vi "sub vi - calibration v2.vi"(6 "Samples":dbl, 8 "Task2":dbl, 9 "Task1":dbl, 10 "Task0":dbl, 11 "Temp Test Cal":dbl) -> ()   [LabVIEW 2017]
uses:
  <vilib>/Platform/TimedLoop/XDataNode/timing_clust.ctl
  <vilib>/Platform/TimedLoop/XDataNode/nitl_modes.ctl
  <vilib>/Platform/TimedLoop/XDataNode/wakeup.ctl
  <vilib>/platform/TimedLoop/XDataNode/XDataNode.xnode
  <vilib>/Platform/TimedLoop/XDataNode/XDNodeRunTimeDep.lvlib
panel:
  out "UPDATE":bool
  in  "stop":bool
  in  "Tab Control":T1(tab)
  out "1-2(TN) Run":dbl
  out "1-2(TL) Run":dbl
  out "1-1(TN) Run":dbl
  out "1-1(TL) Run":dbl
  out "LAB01-1 (GRAPH)":dynamicdata(graph)
  out "LAB01-2 (GRAPH)":dynamicdata(graph)
  in  "LAB01 (CAL)":T2 {"2 (TN) cal" min=0.0 step=0.01 format="%.2f"; "2 (TL) cal" min=0.0 step=0.01 format="%.2f"; "2 (PF) cal" min=0.0 step=0.01 format="%.2f"; "2 (V) cal" min=0.0 step=0.01 format="%.2f"; "2 (A) cal" min=0.0 step=0.01 format="%.2f"; "1 (TN) cal" min=0.0 step=0.01 format="%.2f"; "1 (TL) cal" min=0.0 step=0.01 format="%.2f"; "1 (PF) cal" min=0.0 step=0.01 format="%.2f"; "1 (V) cal" min=0.0 step=0.01 format="%.2f"; "1  (A) cal" min=0.0 step=0.01 format="%.2f"}
  out "LAB01 (SIGNALS)":T3 {"2 (PF)" format="%.2f"; "2 (A)" format="%.1f"; "1 (PF)" format="%.2f"; "1 (A)" format="%.1f"}
  out "2-2(TN) Run":dbl
  out "2-2(TL) Run":dbl
  out "2-1(TN) Run":dbl
  out "2-1(TL) Run":dbl
  out "LAB02 (SIGNALS)":T3 {"2 (PF)" format="%.2f"; "2 (A)" format="%.1f"; "1 (PF)" format="%.2f"; "1 (A)" format="%.1f"}
  in  "LAB02 (CAL)":T4 {"2 (TN) cal" min=0.0 step=0.01 format="%.2f"; "2 (TL) cal" min=0.0 step=0.01 format="%.2f"; "2 (PF) cal" min=0.0 step=0.01 format="%.2f"; "2 (V) cal" min=0.0 step=0.01 format="%.2f"; "2 (A) cal" min=0.0 step=0.01 format="%.2f"; "1 (TN) cal" min=0.0 step=0.01 format="%.2f"; "1 (TL) cal" min=0.0 step=0.01 format="%.2f"; "1 (PF) cal" min=0.0 step=0.01 format="%.2f"; "1 (V) cal" min=0.0 step=0.01 format="%.2f"; "1 (A) cal" min=0.0 step=0.01 format="%.2f"}
  out "LAB02-2 (GRAPH)":dynamicdata(graph)
  out "LAB02-1 (GRAPH)":dynamicdata(graph)
  out "3-2(TN) Run":dbl
  out "3-2(TL) Run":dbl
  out "3-1(TN) Run":dbl
  out "3-1(TL) Run":dbl
  out "LAB03 (SIGNALS)":T3 {"2 (PF)" format="%.2f"; "2 (A)" format="%.1f"; "1 (PF)" format="%.2f"; "1 (A)" format="%.1f"}
  in  "LAB03 (CAL)":T2 {"2 (TN) cal" min=0.0 step=0.01 format="%.2f"; "2 (TL) cal" min=0.0 step=0.01 format="%.2f"; "2 (PF) cal" min=0.0 step=0.01 format="%.2f"; "2 (V) cal" min=0.0 step=0.01 format="%.2f"; "2 (A) cal" min=0.0 step=0.01 format="%.2f"; "1 (TN) cal" min=0.0 step=0.01 format="%.2f"; "1 (TL) cal" min=0.0 step=0.01 format="%.2f"; "1 (PF) cal" min=0.0 step=0.01 format="%.2f"; "1 (V) cal" min=0.0 step=0.01 format="%.2f"; "1  (A) cal" min=0.0 step=0.01 format="%.2f"}
  out "LAB03-2 (GRAPH)":dynamicdata(graph)
  out "LAB03-1 (GRAPH)":dynamicdata(graph)
  out "4-2(TN) Run":dbl
  out "4-2(TL) Run":dbl
  out "4-1(TN) Run":dbl
  out "4-1(TL) Run":dbl
  out "LAB04 (SIGNALS)":T3 {"2 (PF)" format="%.2f"; "2 (A)" format="%.1f"; "1 (PF)" format="%.2f"; "1 (A)" format="%.1f"}
  in  "LAB04 (CAL)":T2 {"2 (TN) cal" min=0.0 step=0.01 format="%.2f"; "2 (TL) cal" min=0.0 step=0.01 format="%.2f"; "2 (PF) cal" min=0.0 step=0.01 format="%.2f"; "2 (V) cal" min=0.0 step=0.01 format="%.2f"; "2 (A) cal" min=0.0 step=0.01 format="%.2f"; "1 (TN) cal" min=0.0 step=0.01 format="%.2f"; "1 (TL) cal" min=0.0 step=0.01 format="%.2f"; "1 (PF) cal" min=0.0 step=0.01 format="%.2f"; "1 (V) cal" min=0.0 step=0.01 format="%.2f"; "1  (A) cal" min=0.0 step=0.01 format="%.2f"}
  out "LAB04-2 (GRAPH)":dynamicdata(graph)
  out "LAB04-1 (GRAPH)":dynamicdata(graph)
  out "5-2(TN) Run":dbl
  out "5-2(TL) Run":dbl
  out "5-1(TN) Run":dbl
  out "5-1(TL) Run":dbl
  out "LAB05 (SIGNALS)":T3 {"2 (PF)" format="%.2f"; "2 (A)" format="%.1f"; "1 (PF)" format="%.2f"; "1 (A)" format="%.1f"}
  in  "LAB05 (CAL)":T2 {"2 (TN) cal" min=0.0 step=0.01 format="%.2f"; "2 (TL) cal" min=0.0 step=0.01 format="%.2f"; "2 (PF) cal" min=0.0 step=0.01 format="%.2f"; "2 (V) cal" min=0.0 step=0.01 format="%.2f"; "2 (A) cal" min=0.0 step=0.01 format="%.2f"; "1 (TN) cal" min=0.0 step=0.01 format="%.2f"; "1 (TL) cal" min=0.0 step=0.01 format="%.2f"; "1 (PF) cal" min=0.0 step=0.01 format="%.2f"; "1 (V) cal" min=0.0 step=0.01 format="%.2f"; "1  (A) cal" min=0.0 step=0.01 format="%.2f"}
  out "LAB05-2 (GRAPH)":dynamicdata(graph)
  out "LAB05-1 (GRAPH)":dynamicdata(graph)
  in  "TEMP REF cal":dbl
  out "AMBIENT TEMP REF":dbl format="%.1f"
  out "Data2":waveform(dbl)[](graph)
  out "Data1":waveform(dbl)[](graph)
  out "Data0":waveform(dbl)[](graph)
  out "Analog Loop Time":dbl
  out "Temperature data error":bool
  out "file error out":errorcluster
  out "AI Error":errorcluster[](array[cluster])
  out "data 0":waveform(dbl)[](array[waveform])
  out "data 1":waveform(dbl)[](array[waveform])
  out "data 2":waveform(dbl)[](array[waveform])
  # "This value is only applied during\ntesting to adjust for insulatred probe\nprofile during current flow temp rise.\nIf any change is made here, make sure\nvalue is changed to same value on\nADM tab."
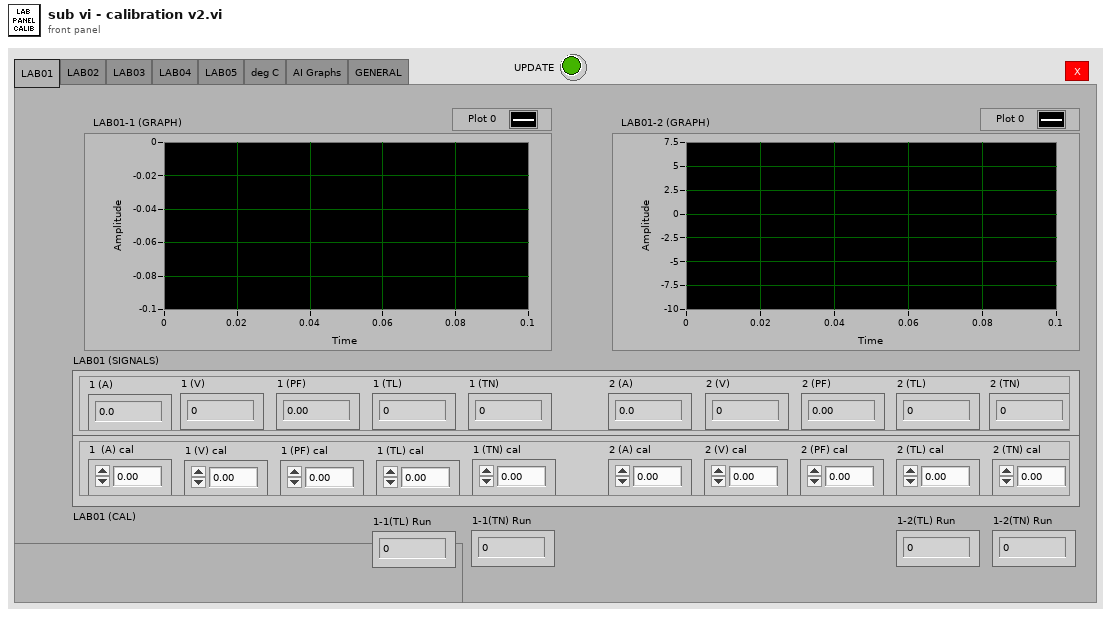
[diagram p1: front panel]
types:
  T1 = enum32{"LAB01", "LAB02", "LAB03", "LAB04", "LAB05", "deg C", "AI Graphs", "GENERAL"}
  T2 = cluster{"1  (A) cal":dbl, "1 (V) cal":dbl, "1 (PF) cal":dbl, "1 (TL) cal":dbl, "1 (TN) cal":dbl, "2 (A) cal":dbl, "2 (V) cal":dbl, "2 (PF) cal":dbl, "2 (TL) cal":dbl, "2 (TN) cal":dbl}
  T3 = cluster{"1 (TL)":dbl, "1 (TN)":dbl, "2 (TL)":dbl, "2 (TN)":dbl, "1 (A)":dbl, "1 (V)":dbl, "1 (PF)":dbl, "2 (A)":dbl, "2 (V)":dbl, "2 (PF)":dbl}
  T4 = cluster{"1 (A) cal":dbl, "1 (V) cal":dbl, "1 (PF) cal":dbl, "1 (TL) cal":dbl, "1 (TN) cal":dbl, "2 (A) cal":dbl, "2 (V) cal":dbl, "2 (PF) cal":dbl, "2 (TL) cal":dbl, "2 (TN) cal":dbl}
  T5 = enum16{"open", "replace", "create", "open or create", "replace or create", "replace or create with confirmation"}
  T6 = typedef "XDNodeRunTimeDep.lvlib/timing_clust.ctl" = cluster{"Expected End [f-1]":u64, "Actual End [f-1]":u64, "Finished Late? [f-1]":bool, "Expected End [i-1]":u64, "Actual End [i-1]":u64, "Finished Late? [i-1]":bool, "Expected Start [i]":u64, "Actual Start [i]":u64, "Expected Start [f]":u64, "Actual Start [f]":u64, "Source Name":string, "Structure Name":string, "Period":i64, "Deadline":i64, "Offset":i64, "Start":i64, "Priority":i32, "Timeout":i32, "Mode":T7, "Wakeup Reason":T8, "Error":errorcluster, "Source Type":string, "Secondary Source Type":string, "Global End Time":u64, "Global Start Time":u64, "Frame Duration":u64, "Iteration Duration":u64, "Assigned CPU":i32, "I/O Scan Engine Mode":u32}
  T7 = typedef "XDNodeRunTimeDep.lvlib/nitl_modes.ctl" = enum32{"No Change", "Process missed periods, maintain original phase", "Discard missed periods, maintain original phase", "Process missed periods, ignore original phase", "Discard missed periods, ignore original phase"}
  T8 = typedef "XDNodeRunTimeDep.lvlib/wakeup.ctl" = enum32{"Normal", "Aborted", "Asynchronous wakeup", "Timing source error", "Timed loop error", "Timeout"}
  T9 = cluster{"LAB01-1 (A)":dbl, "LAB01-1 (V)":dbl, "LAB01-1 (PF)":dbl, "LAB01-2 (A)":dbl, "LAB01-2 (V)":dbl, "LAB01-2 (PF)":dbl}
  T10 = cluster{"LAB02-1 (A)":dbl, "LAB02-1 (V)":dbl, "LAB02-1 (PF)":dbl, "LAB02-2 (A)":dbl, "LAB02-2 (V)":dbl, "LAB02-2 (PF)":dbl}
  T11 = cluster{"LAB03-1 (A)":dbl, "LAB03-1 (V)":dbl, "LAB03-1 (PF)":dbl, "LAB03-2 (A)":dbl, "LAB03-2 (V)":dbl, "LAB03-2 (PF)":dbl}
  T12 = cluster{"LAB04-1 (A)":dbl, "LAB04-1 (V)":dbl, "LAB04-1 (PF)":dbl, "LAB04-2 (A)":dbl, "LAB04-2 (V)":dbl, "LAB04-2 (PF)":dbl}
  T13 = cluster{"LAB05-1 (A)":dbl, "LAB05-1 (V)":dbl, "LAB05-1 (PF)":dbl, "LAB05-2 (A)":dbl, "LAB05-2 (V)":dbl, "LAB05-2 (PF)":dbl}
  T14 = cluster{"T1":dbl, "T2":dbl, "T3":dbl, "T4":dbl, "ID":dbl, "ER":dbl}
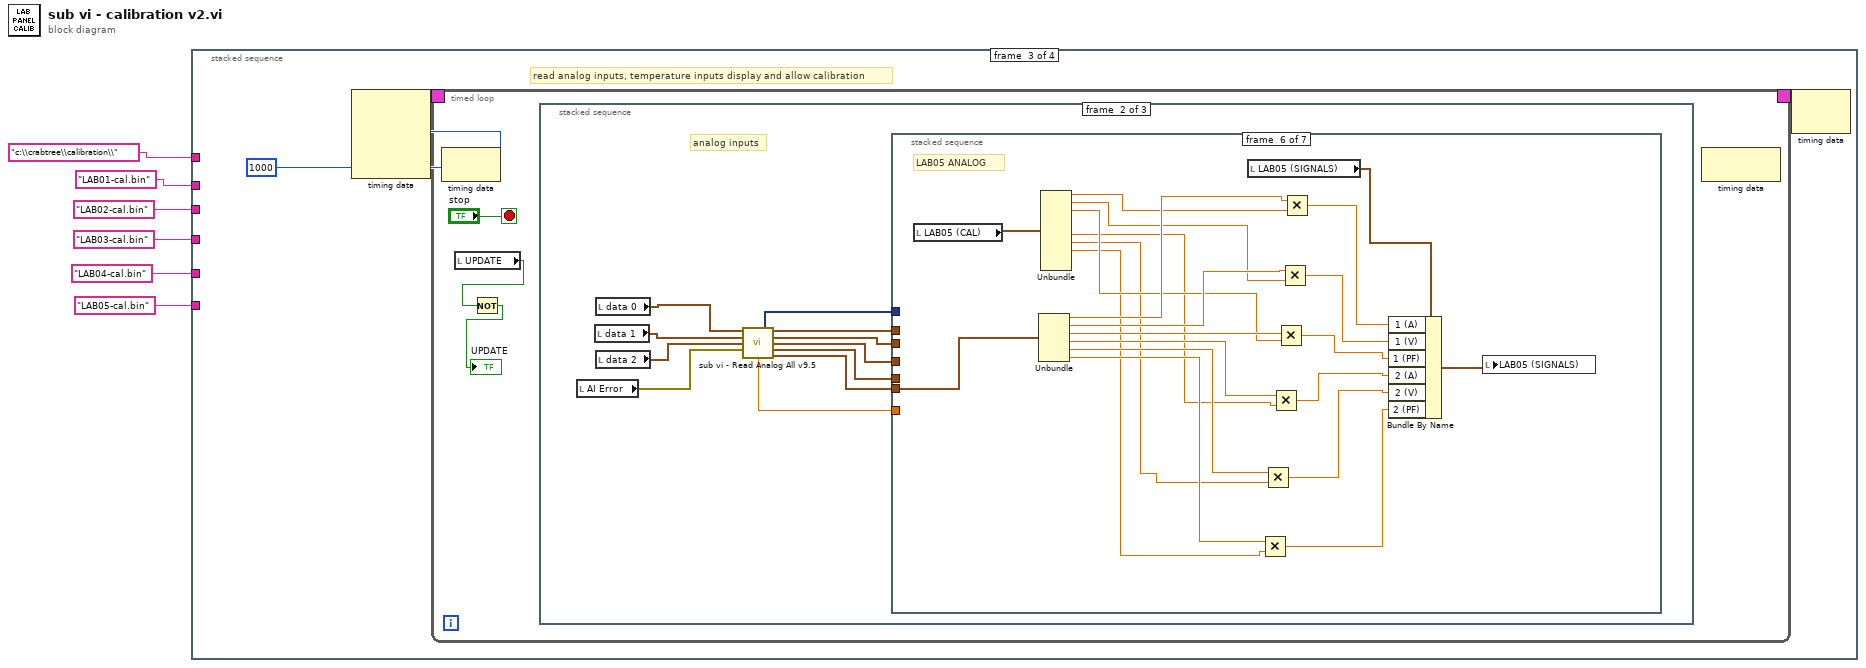
[diagram p0: block diagram]
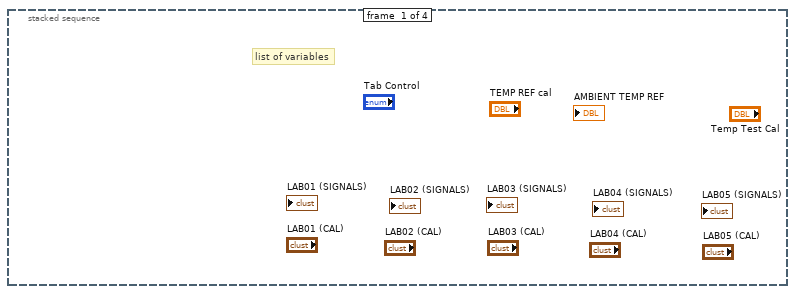
[diagram p2: hidden frame]
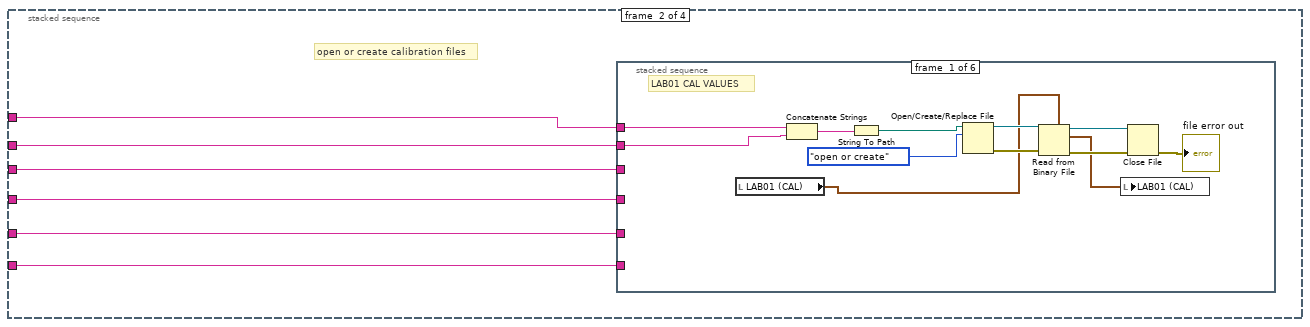
[diagram p3: hidden frame]
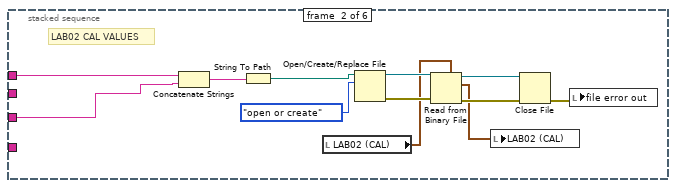
[diagram p4: hidden frame]
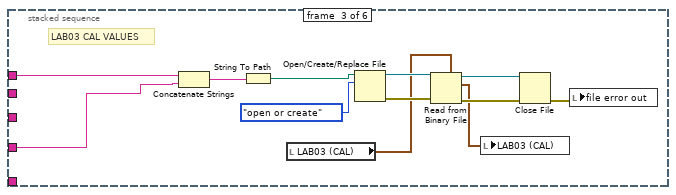
[diagram p5: hidden frame]
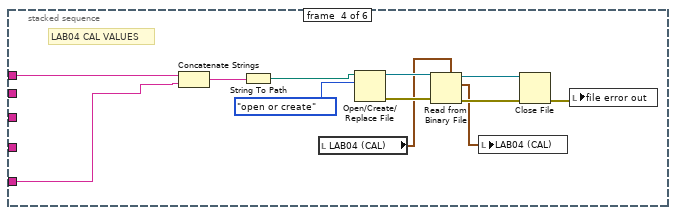
[diagram p6: hidden frame]
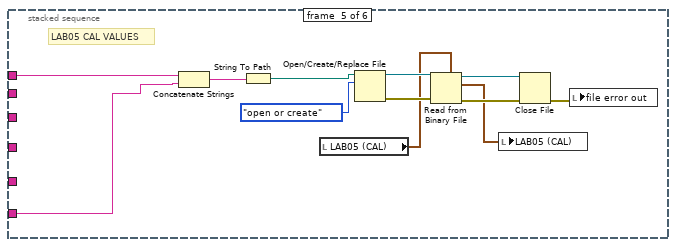
[diagram p7: hidden frame]
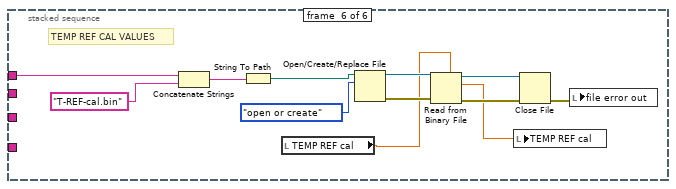
[diagram p8: hidden frame]
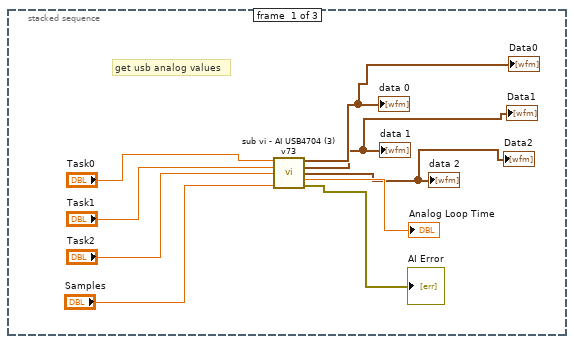
[diagram p9: hidden frame]
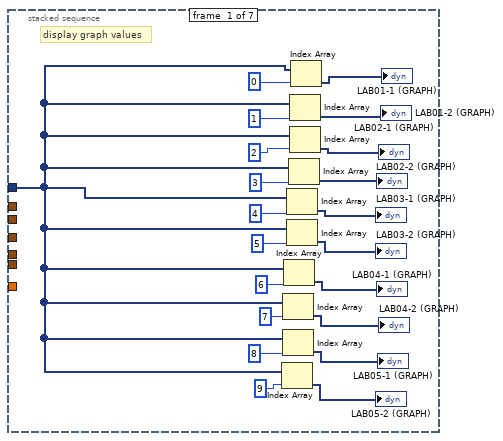
[diagram p10: hidden frame]
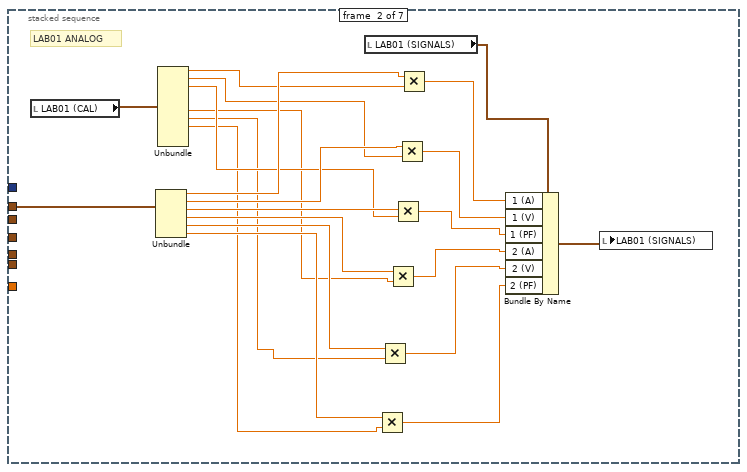
[diagram p11: hidden frame]
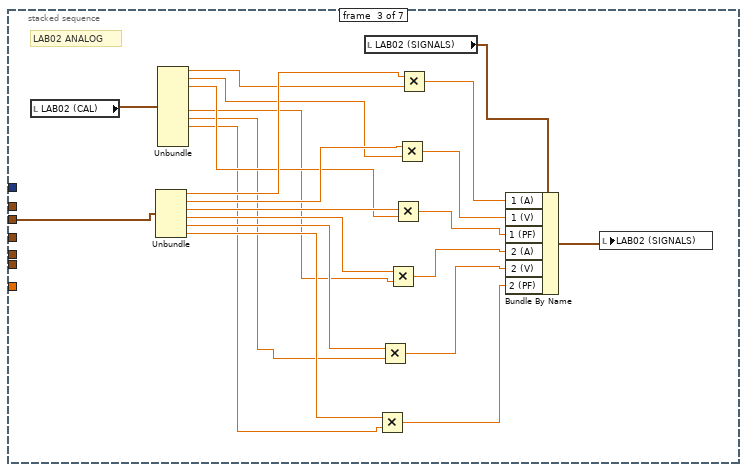
[diagram p12: hidden frame]
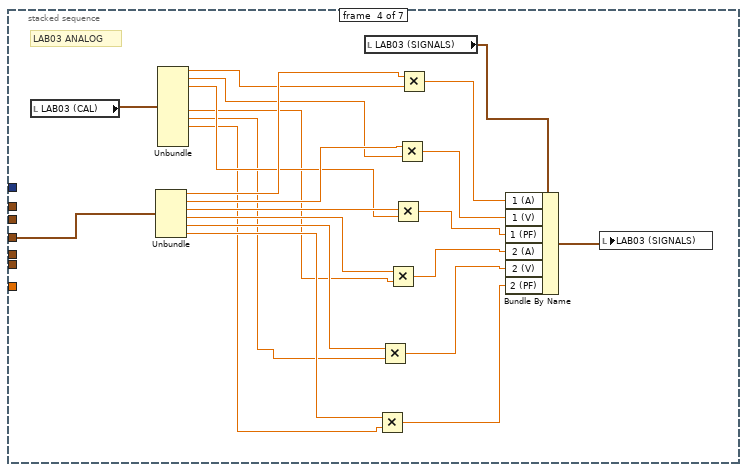
[diagram p13: hidden frame]
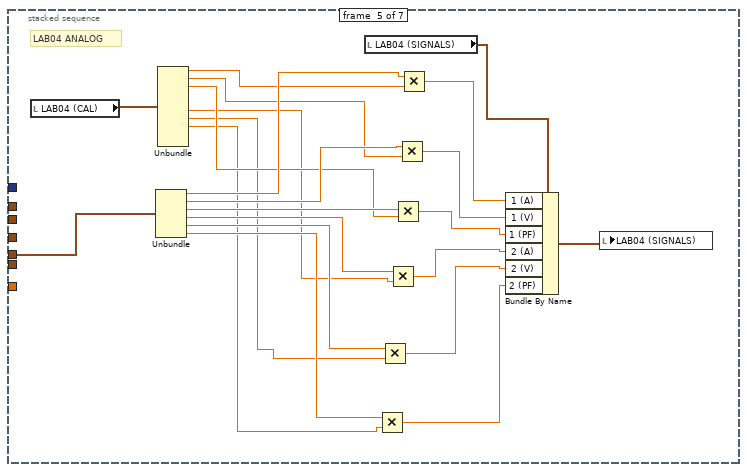
[diagram p14: hidden frame]
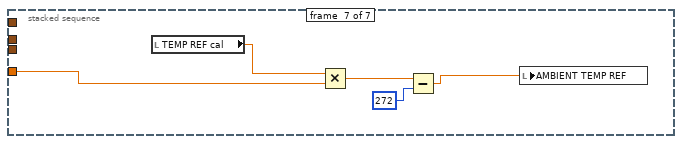
[diagram p15: hidden frame]
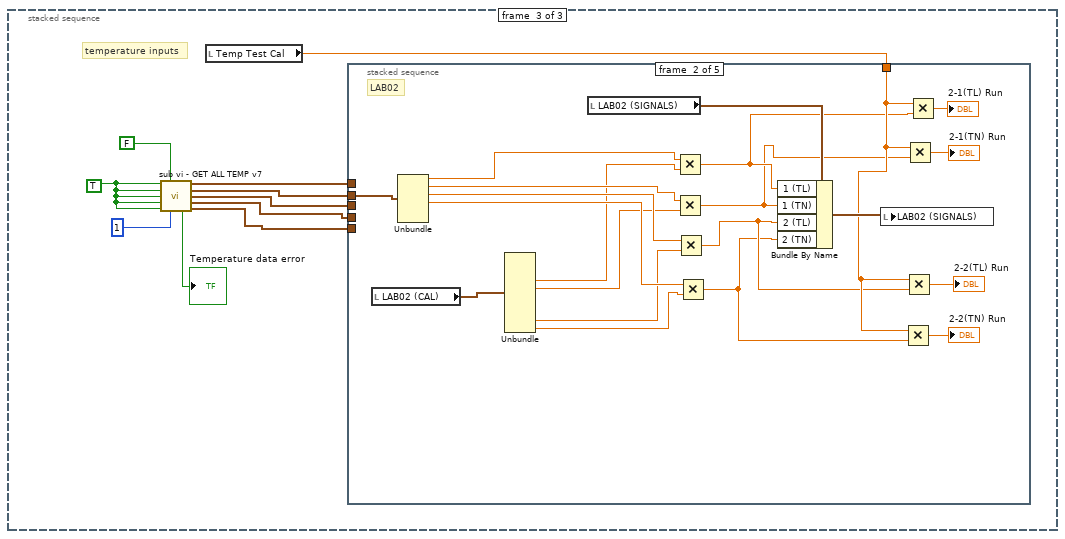
[diagram p16: hidden frame]
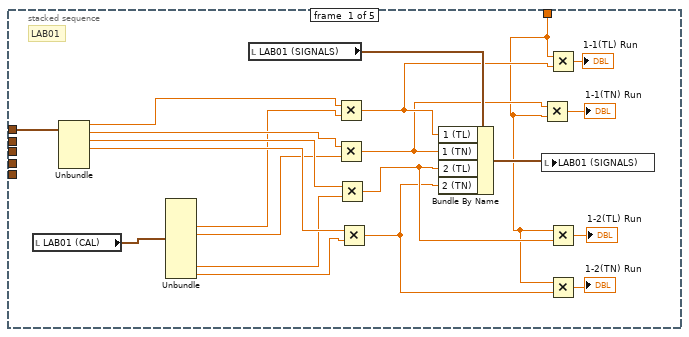
[diagram p17: hidden frame]
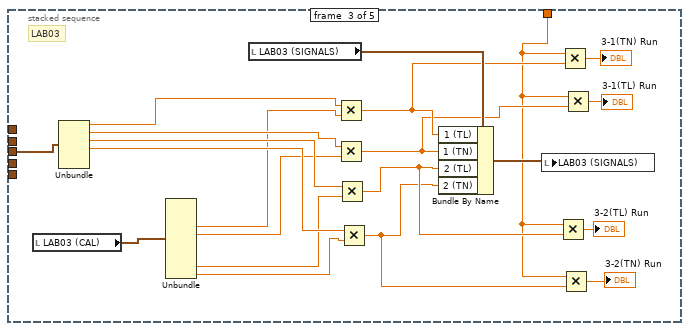
[diagram p18: hidden frame]
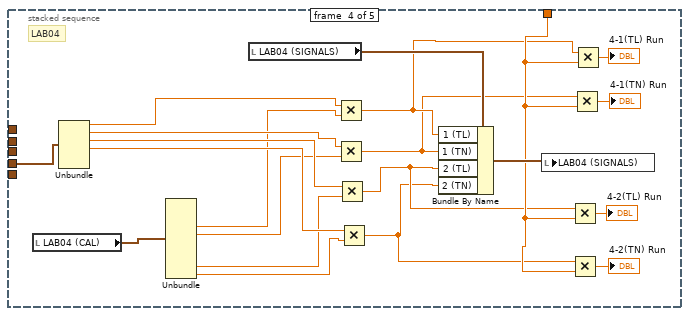
[diagram p19: hidden frame]
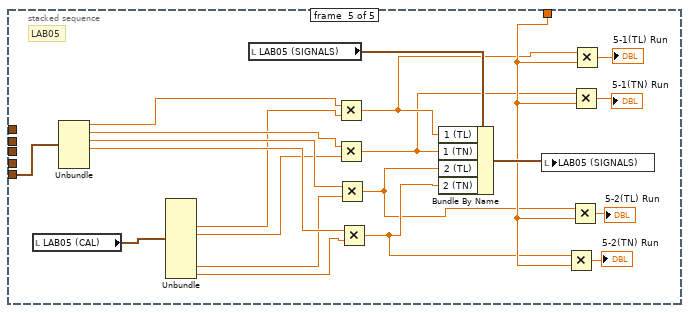
[diagram p20: hidden frame]
diagram:
  n1 = stacked-sequence {
    tunnel: "c:\\crabtree\\calibration\\" -> [_ w12 _ w373]
    tunnel: "LAB01-cal.bin" -> [_ w11 _ w372]
    tunnel: "LAB02-cal.bin" -> [_ w10 _ w371]
    tunnel: "LAB03-cal.bin" -> [_ w9 _ w370]
    tunnel: "LAB04-cal.bin" -> [_ w8 _ w369]
    tunnel: "LAB05-cal.bin" -> [_ w7 _ w368]
    frame #0 {
      # "list of variables"
    }
    frame #1 {
      # "open or create calibration files"
      n2 = stacked-sequence {
        tunnel: w12 -> [w24 w36 w48 w60 w72 w84]
        tunnel: w11 -> [w15 _ _ _ _ _]
        tunnel: w10 -> [_ w27 _ _ _ _]
        tunnel: w9 -> [_ _ w39 _ _ _]
        tunnel: w8 -> [_ _ _ w52 _ _]
        tunnel: w7 -> [_ _ _ _ w63 _]
        frame #0 {
          # "LAB01 CAL VALUES"
          n3 = local read "LAB01 (CAL)"() -> (w14:T2)
          n4 = Concatenate Strings(w24, w15) -> (w23:string)
          n5 = String To Path(string=w23) -> (path=w22:path)
          n6 = Open/Create/Replace File(file path (use dialog)=w22, operation (0:open)=T5."open or create") -> (refnum out=w21:refnum<file>, error out=w20:errorcluster)  [unwired: 4 in, 1 out]
          n7 = Read from Binary File(5:w14, 8:w20, 11:w21) -> (0:w18:errorcluster, 2:w13:T2, 3:w19:refnum<file>)  [unwired: 3 in, 1 out]
          n8 = local write "LAB01 (CAL)"(w13) -> ()
          n9 = Close File(refnum=w19, error in=w18) -> (error out=→"file error out":errorcluster)  [unwired: 1 out]
        }
        frame #1 {
          # "LAB02 CAL VALUES"
          n10 = Concatenate Strings(w36, w27) -> (w35:string)
          n11 = String To Path(string=w35) -> (path=w34:path)
          n12 = local read "LAB02 (CAL)"() -> (w26:T4)
          n13 = Open/Create/Replace File(file path (use dialog)=w34, operation (0:open)=T5."open or create") -> (refnum out=w33:refnum<file>, error out=w32:errorcluster)  [unwired: 4 in, 1 out]
          n14 = Read from Binary File(5:w26, 8:w32, 11:w33) -> (0:w30:errorcluster, 2:w25:T4, 3:w31:refnum<file>)  [unwired: 3 in, 1 out]
          n15 = local write "LAB02 (CAL)"(w25) -> ()
          n16 = Close File(refnum=w31, error in=w30) -> (error out=w28:errorcluster)  [unwired: 1 out]
          n17 = local write "file error out"(w28) -> ()
        }
        frame #2 {
          # "LAB03 CAL VALUES"
          n18 = Concatenate Strings(w48, w39) -> (w47:string)
          n19 = String To Path(string=w47) -> (path=w46:path)
          n20 = local read "LAB03 (CAL)"() -> (w38:T2)
          n21 = Open/Create/Replace File(file path (use dialog)=w46, operation (0:open)=T5."open or create") -> (refnum out=w45:refnum<file>, error out=w44:errorcluster)  [unwired: 4 in, 1 out]
          n22 = Read from Binary File(5:w38, 8:w44, 11:w45) -> (0:w42:errorcluster, 2:w37:T2, 3:w43:refnum<file>)  [unwired: 3 in, 1 out]
          n23 = local write "LAB03 (CAL)"(w37) -> ()
          n24 = Close File(refnum=w43, error in=w42) -> (error out=w40:errorcluster)  [unwired: 1 out]
          n25 = local write "file error out"(w40) -> ()
        }
        frame #3 {
          # "LAB04 CAL VALUES"
          n26 = Concatenate Strings(w60, w52) -> (w59:string)
          n27 = String To Path(string=w59) -> (path=w58:path)
          n28 = local read "LAB04 (CAL)"() -> (w50:T2)
          n29 = Open/Create/Replace File(file path (use dialog)=w58, operation (0:open)=T5."open or create") -> (refnum out=w57:refnum<file>, error out=w56:errorcluster)  [unwired: 4 in, 1 out]
          n30 = Read from Binary File(5:w50, 8:w56, 11:w57) -> (0:w54:errorcluster, 2:w49:T2, 3:w55:refnum<file>)  [unwired: 3 in, 1 out]
          n31 = local write "LAB04 (CAL)"(w49) -> ()
          n32 = Close File(refnum=w55, error in=w54) -> (error out=w53:errorcluster)  [unwired: 1 out]
          n33 = local write "file error out"(w53) -> ()
        }
        frame #4 {
          # "LAB05 CAL VALUES"
          n34 = Concatenate Strings(w72, w63) -> (w71:string)
          n35 = String To Path(string=w71) -> (path=w70:path)
          n36 = local read "LAB05 (CAL)"() -> (w62:T2)
          n37 = Open/Create/Replace File(file path (use dialog)=w70, operation (0:open)=T5."open or create") -> (refnum out=w69:refnum<file>, error out=w68:errorcluster)  [unwired: 4 in, 1 out]
          n38 = Read from Binary File(5:w62, 8:w68, 11:w69) -> (0:w66:errorcluster, 2:w61:T2, 3:w67:refnum<file>)  [unwired: 3 in, 1 out]
          n39 = local write "LAB05 (CAL)"(w61) -> ()
          n40 = Close File(refnum=w67, error in=w66) -> (error out=w64:errorcluster)  [unwired: 1 out]
          n41 = local write "file error out"(w64) -> ()
        }
        frame #5 {
          # "TEMP REF CAL VALUES"
          n42 = Concatenate Strings(w84, "T-REF-cal.bin") -> (w83:string)
          n43 = String To Path(string=w83) -> (path=w82:path)
          n44 = local read "TEMP REF cal"() -> (w74:dbl)
          n45 = Open/Create/Replace File(file path (use dialog)=w82, operation (0:open)=T5."open or create") -> (refnum out=w81:refnum<file>, error out=w80:errorcluster)  [unwired: 4 in, 1 out]
          n46 = Read from Binary File(5:w74, 8:w80, 11:w81) -> (0:w78:errorcluster, 2:w73:dbl, 3:w79:refnum<file>)  [unwired: 3 in, 1 out]
          n47 = local write "TEMP REF cal"(w73) -> ()
          n48 = Close File(refnum=w79, error in=w78) -> (error out=w76:errorcluster)  [unwired: 1 out]
          n49 = local write "file error out"(w76) -> ()
        }
      }
    }
    frame #2 {
      # "read analog inputs, temperature inputs display and allow calibration"
      n50 = node-c288(1000) -> (w87:T6)  [unwired: 3 in]
      n51 = timed-loop {
        timing: w87 -> [_]
        timing-out: [_] -> w86
        stop <- "stop" stop-if-true
        n52 = node-c288() -> ()  [unwired: 1 in, 1 out]
        n53 = local read "UPDATE"() -> (w88:bool)
        n54 = Not(x=w88) -> (.not. x?=→"UPDATE":bool)
        n55 = stacked-sequence {
          frame #0 {
            # "get usb analog values"
            n56 = call "sub vi - AI USB4704 (3) v73.vi"("Task0"="Task0", "Task1"="Task1", "Task2"="Task2", "SAMPLES"="Samples") -> ("data 0"=→"data 0" →"Data0":waveform(dbl)[], "data 1"=→"data 1" →"Data1":waveform(dbl)[], "data 2"=→"data 2" →"Data2":waveform(dbl)[], "loop time"=→"Analog Loop Time":dbl, "error array"=→"AI Error":errorcluster[])  [unwired: 7 in]
          }
          frame #1 {
            # "analog inputs"
            n57 = local read "AI Error"() -> (w100:errorcluster[])
            n58 = local read "data 1"() -> (w102:waveform(dbl)[])
            n59 = local read "data 0"() -> (w103:waveform(dbl)[])
            n60 = local read "data 2"() -> (w101:waveform(dbl)[])
            n61 = call "sub vi - Read Analog All v9.5.vi"("data 0"=w103, "data 1"=w102, "data 2"=w101, "AI Error"=w100) -> ("array GRAPH"=w110:dynamicdata[], "LAB01"=w109:T9, "LAB02"=w108:T10, "LAB03"=w107:T11, "LAB04"=w106:T12, "deg C"=w104:dbl, "LAB05"=w105:T13)  [unwired: 4 in, 1 out]
            n62 = stacked-sequence {
              tunnel: w110 -> [w130 _ _ _ _ _ _]
              tunnel: w109 -> [_ w152 _ _ _ _ _]
              tunnel: w107 -> [_ _ _ w176 _ _ _]
              tunnel: w108 -> [_ _ w154 _ _ _ _]
              tunnel: w106 -> [_ _ _ _ w198 _ _]
              tunnel: w105 -> [_ _ _ _ _ w220 _]
              tunnel: w104 -> [_ _ _ _ _ _ w245]
              frame #0 {
                # "display graph values"
                n63 = Index Array(array=w130, index=9) -> (element=→"LAB05-2 (GRAPH)":dynamicdata)
                n64 = Index Array(array=w130, index=7) -> (element=→"LAB04-2 (GRAPH)":dynamicdata)
                n65 = Index Array(array=w130, index=8) -> (element=→"LAB05-1 (GRAPH)":dynamicdata)
                n66 = Index Array(array=w130, index=6) -> (element=→"LAB04-1 (GRAPH)":dynamicdata)
                n67 = Index Array(array=w130, index=4) -> (element=→"LAB03-1 (GRAPH)":dynamicdata)
                n68 = Index Array(array=w130, index=5) -> (element=→"LAB03-2 (GRAPH)":dynamicdata)
                n69 = Index Array(array=w130, index=3) -> (element=→"LAB02-2 (GRAPH)":dynamicdata)
                n70 = Index Array(array=w130, index=1) -> (element=→"LAB01-2 (GRAPH)":dynamicdata)
                n71 = Index Array(array=w130, index=2) -> (element=→"LAB02-1 (GRAPH)":dynamicdata)
                n72 = Index Array(array=w130, index=0) -> (element=→"LAB01-1 (GRAPH)":dynamicdata)
              }
              frame #1 {
                # "LAB01 ANALOG"
                n73 = local read "LAB01 (CAL)"() -> (w153:T2)
                n74 = Unbundle(w152) -> ("LAB01-1 (A)"=w151:dbl, "LAB01-1 (V)"=w150:dbl, "LAB01-1 (PF)"=w149:dbl, "LAB01-2 (A)"=w148:dbl, "LAB01-2 (V)"=w147:dbl, "LAB01-2 (PF)"=w146:dbl)
                n75 = Unbundle(w153) -> ("1  (A) cal"=w145:dbl, "1 (V) cal"=w144:dbl, "1 (PF) cal"=w143:dbl, "2 (A) cal"=w142:dbl, "2 (V) cal"=w141:dbl, "2 (PF) cal"=w140:dbl)  [unwired: 4 out]
                n76 = local read "LAB01 (SIGNALS)"() -> (w139:T3)
                n77 = Multiply(x=w146, y=w140) -> (x*y=w133:dbl)
                n78 = Multiply(x=w147, y=w141) -> (x*y=w134:dbl)
                n79 = Multiply(x=w148, y=w142) -> (x*y=w135:dbl)
                n80 = Multiply(x=w149, y=w143) -> (x*y=w136:dbl)
                n81 = Multiply(x=w150, y=w144) -> (x*y=w137:dbl)
                n82 = Multiply(x=w151, y=w145) -> (x*y=w138:dbl)
                n83 = Bundle By Name(cluster=w139, "1 (A)"=w138, "1 (V)"=w137, "1 (PF)"=w136, "2 (A)"=w135, "2 (V)"=w134, "2 (PF)"=w133) -> (w132:T3)
                n84 = local write "LAB01 (SIGNALS)"(w132) -> ()
              }
              frame #2 {
                # "LAB02 ANALOG"
                n85 = local read "LAB02 (CAL)"() -> (w175:T4)
                n86 = Unbundle(w154) -> ("LAB02-1 (A)"=w174:dbl, "LAB02-1 (V)"=w173:dbl, "LAB02-1 (PF)"=w172:dbl, "LAB02-2 (A)"=w171:dbl, "LAB02-2 (V)"=w170:dbl, "LAB02-2 (PF)"=w169:dbl)
                n87 = Unbundle(w175) -> ("1 (A) cal"=w168:dbl, "1 (V) cal"=w167:dbl, "1 (PF) cal"=w166:dbl, "2 (A) cal"=w165:dbl, "2 (V) cal"=w164:dbl, "2 (PF) cal"=w163:dbl)  [unwired: 4 out]
                n88 = local read "LAB02 (SIGNALS)"() -> (w162:T3)
                n89 = Multiply(x=w169, y=w163) -> (x*y=w156:dbl)
                n90 = Multiply(x=w170, y=w164) -> (x*y=w157:dbl)
                n91 = Multiply(x=w171, y=w165) -> (x*y=w158:dbl)
                n92 = Multiply(x=w172, y=w166) -> (x*y=w159:dbl)
                n93 = Multiply(x=w173, y=w167) -> (x*y=w160:dbl)
                n94 = Multiply(x=w174, y=w168) -> (x*y=w161:dbl)
                n95 = Bundle By Name(cluster=w162, "1 (A)"=w161, "1 (V)"=w160, "1 (PF)"=w159, "2 (A)"=w158, "2 (V)"=w157, "2 (PF)"=w156) -> (w155:T3)
                n96 = local write "LAB02 (SIGNALS)"(w155) -> ()
              }
              frame #3 {
                # "LAB03 ANALOG"
                n97 = local read "LAB03 (CAL)"() -> (w197:T2)
                n98 = Unbundle(w176) -> ("LAB03-1 (A)"=w196:dbl, "LAB03-1 (V)"=w195:dbl, "LAB03-1 (PF)"=w194:dbl, "LAB03-2 (A)"=w193:dbl, "LAB03-2 (V)"=w192:dbl, "LAB03-2 (PF)"=w191:dbl)
                n99 = Unbundle(w197) -> ("1  (A) cal"=w190:dbl, "1 (V) cal"=w189:dbl, "1 (PF) cal"=w188:dbl, "2 (A) cal"=w187:dbl, "2 (V) cal"=w186:dbl, "2 (PF) cal"=w185:dbl)  [unwired: 4 out]
                n100 = local read "LAB03 (SIGNALS)"() -> (w184:T3)
                n101 = Multiply(x=w191, y=w185) -> (x*y=w178:dbl)
                n102 = Multiply(x=w192, y=w186) -> (x*y=w179:dbl)
                n103 = Multiply(x=w193, y=w187) -> (x*y=w180:dbl)
                n104 = Multiply(x=w194, y=w188) -> (x*y=w181:dbl)
                n105 = Multiply(x=w195, y=w189) -> (x*y=w182:dbl)
                n106 = Multiply(x=w196, y=w190) -> (x*y=w183:dbl)
                n107 = Bundle By Name(cluster=w184, "1 (A)"=w183, "1 (V)"=w182, "1 (PF)"=w181, "2 (A)"=w180, "2 (V)"=w179, "2 (PF)"=w178) -> (w177:T3)
                n108 = local write "LAB03 (SIGNALS)"(w177) -> ()
              }
              frame #4 {
                # "LAB04 ANALOG"
                n109 = local read "LAB04 (CAL)"() -> (w219:T2)
                n110 = Unbundle(w198) -> ("LAB04-1 (A)"=w218:dbl, "LAB04-1 (V)"=w217:dbl, "LAB04-1 (PF)"=w216:dbl, "LAB04-2 (A)"=w215:dbl, "LAB04-2 (V)"=w214:dbl, "LAB04-2 (PF)"=w213:dbl)
                n111 = Unbundle(w219) -> ("1  (A) cal"=w212:dbl, "1 (V) cal"=w211:dbl, "1 (PF) cal"=w210:dbl, "2 (A) cal"=w209:dbl, "2 (V) cal"=w208:dbl, "2 (PF) cal"=w207:dbl)  [unwired: 4 out]
                n112 = local read "LAB04 (SIGNALS)"() -> (w206:T3)
                n113 = Multiply(x=w213, y=w207) -> (x*y=w200:dbl)
                n114 = Multiply(x=w214, y=w208) -> (x*y=w201:dbl)
                n115 = Multiply(x=w215, y=w209) -> (x*y=w202:dbl)
                n116 = Multiply(x=w216, y=w210) -> (x*y=w203:dbl)
                n117 = Multiply(x=w217, y=w211) -> (x*y=w204:dbl)
                n118 = Multiply(x=w218, y=w212) -> (x*y=w205:dbl)
                n119 = Bundle By Name(cluster=w206, "1 (A)"=w205, "1 (V)"=w204, "1 (PF)"=w203, "2 (A)"=w202, "2 (V)"=w201, "2 (PF)"=w200) -> (w199:T3)
                n120 = local write "LAB04 (SIGNALS)"(w199) -> ()
              }
              frame #5 {
                # "LAB05 ANALOG"
                n121 = local read "LAB05 (CAL)"() -> (w241:T2)
                n122 = Unbundle(w220) -> ("LAB05-1 (A)"=w240:dbl, "LAB05-1 (V)"=w239:dbl, "LAB05-1 (PF)"=w238:dbl, "LAB05-2 (A)"=w237:dbl, "LAB05-2 (V)"=w236:dbl, "LAB05-2 (PF)"=w235:dbl)
                n123 = Unbundle(w241) -> ("1  (A) cal"=w234:dbl, "1 (V) cal"=w233:dbl, "1 (PF) cal"=w232:dbl, "2 (A) cal"=w231:dbl, "2 (V) cal"=w230:dbl, "2 (PF) cal"=w229:dbl)  [unwired: 4 out]
                n124 = local read "LAB05 (SIGNALS)"() -> (w228:T3)
                n125 = Multiply(x=w235, y=w229) -> (x*y=w222:dbl)
                n126 = Multiply(x=w236, y=w230) -> (x*y=w223:dbl)
                n127 = Multiply(x=w237, y=w231) -> (x*y=w224:dbl)
                n128 = Multiply(x=w238, y=w232) -> (x*y=w225:dbl)
                n129 = Multiply(x=w239, y=w233) -> (x*y=w226:dbl)
                n130 = Multiply(x=w240, y=w234) -> (x*y=w227:dbl)
                n131 = Bundle By Name(cluster=w228, "1 (A)"=w227, "1 (V)"=w226, "1 (PF)"=w225, "2 (A)"=w224, "2 (V)"=w223, "2 (PF)"=w222) -> (w221:T3)
                n132 = local write "LAB05 (SIGNALS)"(w221) -> ()
              }
              frame #6 {
                n133 = local read "TEMP REF cal"() -> (w246:dbl)
                n134 = Multiply(x=w246, y=w245) -> (x*y=w244:dbl)
                n135 = Subtract(x=w244, y=272) -> (x-y=w242:dbl)
                n136 = local write "AMBIENT TEMP REF"(w242) -> ()
              }
            }
          }
          frame #2 {
            w256 = TRUE
            # "temperature inputs"
            n137 = call "sub vi - GET ALL TEMP v7.vi"("LA01-EN"=w256, "simulate"=FALSE, "LA02-EN"=w256, "LA03-EN"=w256, "LA04-EN"=w256, "LA05-EN"=w256, "Gen Cal Value"=1) -> ("LA01 TEMP"=w254:T14, "LA02 TEMP"=w252:T14, "LA03 TEMP"=w251:T14, "LA04 TEMP"=w250:T14, "error"=→"Temperature data error":bool, "LA05 TEMP"=w249:T14)  [unwired: 3 out]
            n138 = local read "Temp Test Cal"() -> (w247:dbl)
            n139 = stacked-sequence {
              tunnel: w254 -> [w276 _ _ _ _]
              tunnel: w252 -> [_ w287 _ _ _]
              tunnel: w251 -> [_ _ w308 _ _]
              tunnel: w250 -> [_ _ _ w329 _]
              tunnel: w249 -> [_ _ _ _ w350]
              tunnel: w247 -> [w257 w282 w300 w324 w345]
              frame #0 {
                # "LAB01"
                n140 = local read "LAB01 (CAL)"() -> (w277:T2)
                n141 = Unbundle(w276) -> ("T1"=w275:dbl, "T2"=w274:dbl, "T3"=w273:dbl, "T4"=w272:dbl)  [unwired: 2 out]
                n142 = Unbundle(w277) -> ("1 (TL) cal"=w271:dbl, "1 (TN) cal"=w270:dbl, "2 (TL) cal"=w269:dbl, "2 (TN) cal"=w268:dbl)  [unwired: 6 out]
                n143 = local read "LAB01 (SIGNALS)"() -> (w267:T3)
                n144 = Multiply(x=w275, y=w271) -> (x*y=w264:dbl)
                n145 = Multiply(x=w274, y=w270) -> (x*y=w262:dbl)
                n146 = Multiply(x=w273, y=w269) -> (x*y=w259:dbl)
                n147 = Multiply(x=w272, y=w268) -> (x*y=w258:dbl)
                n148 = Bundle By Name(cluster=w267, "1 (TL)"=w264, "1 (TN)"=w262, "2 (TL)"=w259, "2 (TN)"=w258) -> (w266:T3)
                n149 = Multiply(x=w262, y=w257) -> (x*y=→"1-1(TN) Run":dbl)
                n150 = local write "LAB01 (SIGNALS)"(w266) -> ()
                n151 = Multiply(x=w257, y=w264) -> (x*y=→"1-1(TL) Run":dbl)
                n152 = Multiply(x=w257, y=w259) -> (x*y=→"1-2(TL) Run":dbl)
                n153 = Multiply(x=w257, y=w258) -> (x*y=→"1-2(TN) Run":dbl)
              }
              frame #1 {
                # "LAB02"
                n154 = local read "LAB02 (CAL)"() -> (w298:T4)
                n155 = Unbundle(w287) -> ("T1"=w297:dbl, "T2"=w296:dbl, "T3"=w295:dbl, "T4"=w294:dbl)  [unwired: 2 out]
                n156 = Unbundle(w298) -> ("1 (TL) cal"=w293:dbl, "1 (TN) cal"=w292:dbl, "2 (TL) cal"=w291:dbl, "2 (TN) cal"=w290:dbl)  [unwired: 6 out]
                n157 = local read "LAB02 (SIGNALS)"() -> (w289:T3)
                n158 = Multiply(x=w297, y=w293) -> (x*y=w281:dbl)
                n159 = Multiply(x=w296, y=w292) -> (x*y=w280:dbl)
                n160 = Multiply(x=w295, y=w291) -> (x*y=w279:dbl)
                n161 = Multiply(x=w294, y=w290) -> (x*y=w278:dbl)
                n162 = Bundle By Name(cluster=w289, "1 (TL)"=w281, "1 (TN)"=w280, "2 (TL)"=w279, "2 (TN)"=w278) -> (w288:T3)
                n163 = local write "LAB02 (SIGNALS)"(w288) -> ()
                n164 = Multiply(x=w282, y=w278) -> (x*y=→"2-2(TN) Run":dbl)
                n165 = Multiply(x=w282, y=w279) -> (x*y=→"2-2(TL) Run":dbl)
                n166 = Multiply(x=w282, y=w280) -> (x*y=→"2-1(TN) Run":dbl)
                n167 = Multiply(x=w282, y=w281) -> (x*y=→"2-1(TL) Run":dbl)
              }
              frame #2 {
                # "LAB03"
                n168 = local read "LAB03 (CAL)"() -> (w319:T2)
                n169 = Unbundle(w308) -> ("T1"=w318:dbl, "T2"=w317:dbl, "T3"=w316:dbl, "T4"=w315:dbl)  [unwired: 2 out]
                n170 = Unbundle(w319) -> ("1 (TL) cal"=w314:dbl, "1 (TN) cal"=w313:dbl, "2 (TL) cal"=w312:dbl, "2 (TN) cal"=w311:dbl)  [unwired: 6 out]
                n171 = local read "LAB03 (SIGNALS)"() -> (w310:T3)
                n172 = Multiply(x=w318, y=w314) -> (x*y=w304:dbl)
                n173 = Multiply(x=w317, y=w313) -> (x*y=w303:dbl)
                n174 = Multiply(x=w316, y=w312) -> (x*y=w302:dbl)
                n175 = Multiply(x=w315, y=w311) -> (x*y=w301:dbl)
                n176 = Bundle By Name(cluster=w310, "1 (TL)"=w304, "1 (TN)"=w303, "2 (TL)"=w302, "2 (TN)"=w301) -> (w309:T3)
                n177 = local write "LAB03 (SIGNALS)"(w309) -> ()
                n178 = Multiply(x=w300, y=w302) -> (x*y=→"3-2(TL) Run":dbl)
                n179 = Multiply(x=w300, y=w304) -> (x*y=→"3-1(TN) Run":dbl)
                n180 = Multiply(x=w300, y=w301) -> (x*y=→"3-2(TN) Run":dbl)
                n181 = Multiply(x=w300, y=w303) -> (x*y=→"3-1(TL) Run":dbl)
              }
              frame #3 {
                # "LAB04"
                n182 = local read "LAB04 (CAL)"() -> (w340:T2)
                n183 = Unbundle(w329) -> ("T1"=w339:dbl, "T2"=w338:dbl, "T3"=w337:dbl, "T4"=w336:dbl)  [unwired: 2 out]
                n184 = Unbundle(w340) -> ("1 (TL) cal"=w335:dbl, "1 (TN) cal"=w334:dbl, "2 (TL) cal"=w333:dbl, "2 (TN) cal"=w332:dbl)  [unwired: 6 out]
                n185 = local read "LAB04 (SIGNALS)"() -> (w331:T3)
                n186 = Multiply(x=w339, y=w335) -> (x*y=w323:dbl)
                n187 = Multiply(x=w338, y=w334) -> (x*y=w322:dbl)
                n188 = Multiply(x=w337, y=w333) -> (x*y=w321:dbl)
                n189 = Multiply(x=w336, y=w332) -> (x*y=w320:dbl)
                n190 = Bundle By Name(cluster=w331, "1 (TL)"=w323, "1 (TN)"=w322, "2 (TL)"=w321, "2 (TN)"=w320) -> (w330:T3)
                n191 = local write "LAB04 (SIGNALS)"(w330) -> ()
                n192 = Multiply(x=w321, y=w324) -> (x*y=→"4-2(TL) Run":dbl)
                n193 = Multiply(x=w320, y=w324) -> (x*y=→"4-2(TN) Run":dbl)
                n194 = Multiply(x=w322, y=w324) -> (x*y=→"4-1(TN) Run":dbl)
                n195 = Multiply(x=w323, y=w324) -> (x*y=→"4-1(TL) Run":dbl)
              }
              frame #4 {
                # "LAB05"
                n196 = local read "LAB05 (CAL)"() -> (w361:T2)
                n197 = Unbundle(w350) -> ("T1"=w360:dbl, "T2"=w359:dbl, "T3"=w358:dbl, "T4"=w357:dbl)  [unwired: 2 out]
                n198 = Unbundle(w361) -> ("1 (TL) cal"=w356:dbl, "1 (TN) cal"=w355:dbl, "2 (TL) cal"=w354:dbl, "2 (TN) cal"=w353:dbl)  [unwired: 6 out]
                n199 = local read "LAB05 (SIGNALS)"() -> (w352:T3)
                n200 = Multiply(x=w360, y=w356) -> (x*y=w344:dbl)
                n201 = Multiply(x=w359, y=w355) -> (x*y=w343:dbl)
                n202 = Multiply(x=w358, y=w354) -> (x*y=w341:dbl)
                n203 = Multiply(x=w357, y=w353) -> (x*y=w342:dbl)
                n204 = Bundle By Name(cluster=w352, "1 (TL)"=w344, "1 (TN)"=w343, "2 (TL)"=w341, "2 (TN)"=w342) -> (w351:T3)
                n205 = local write "LAB05 (SIGNALS)"(w351) -> ()
                n206 = Multiply(x=w342, y=w345) -> (x*y=→"5-2(TN) Run":dbl)
                n207 = Multiply(x=w341, y=w345) -> (x*y=→"5-2(TL) Run":dbl)
                n208 = Multiply(x=w343, y=w345) -> (x*y=→"5-1(TN) Run":dbl)
                n209 = Multiply(x=w344, y=w345) -> (x*y=→"5-1(TL) Run":dbl)
              }
            }
          }
        }
        n210 = node-c288() -> ()  [unwired: 1 in, 1 out]
      }
      n211 = node-c288(w86) -> ()  [unwired: 1 out]
    }
    frame #3 {
      # "save all calibration data"
      n212 = stacked-sequence {
        tunnel: w373 -> [w383 w394 w405 w416 w427 w438]
        tunnel: w372 -> [w382 _ _ _ _ _]
        tunnel: w371 -> [_ w385 _ _ _ _]
        tunnel: w370 -> [_ _ w396 _ _ _]
        tunnel: w369 -> [_ _ _ w407 _ _]
        tunnel: w368 -> [_ _ _ _ w418 _]
        frame #0 {
          # "LAB01"
          n213 = Concatenate Strings(w383, w382) -> (w384:string)
          n214 = String To Path(string=w384) -> (path=w381:path)
          n215 = Open/Create/Replace File(file path (use dialog)=w381, operation (0:open)=4) -> (refnum out=w380:refnum<file>, error out=w379:errorcluster)  [unwired: 4 in, 1 out]
          n216 = local read "LAB01 (CAL)"() -> (w374:T2)
          n217 = Write to Binary File(file (use dialog)=w380, data=w374, error in=w379) -> (refnum out=w378:refnum<file>, error out=w377:errorcluster)  [unwired: 3 in, 1 out]
          n218 = Close File(refnum=w378, error in=w377) -> (error out=w376:errorcluster)  [unwired: 1 out]
          n219 = local write "file error out"(w376) -> ()
        }
        frame #1 {
          # "LAB02"
          n220 = Concatenate Strings(w394, w385) -> (w395:string)
          n221 = String To Path(string=w395) -> (path=w393:path)
          n222 = Open/Create/Replace File(file path (use dialog)=w393, operation (0:open)=4) -> (refnum out=w392:refnum<file>, error out=w391:errorcluster)  [unwired: 4 in, 1 out]
          n223 = local read "LAB02 (CAL)"() -> (w386:T4)
          n224 = Write to Binary File(file (use dialog)=w392, data=w386, error in=w391) -> (refnum out=w390:refnum<file>, error out=w389:errorcluster)  [unwired: 3 in, 1 out]
          n225 = Close File(refnum=w390, error in=w389) -> (error out=w388:errorcluster)  [unwired: 1 out]
          n226 = local write "file error out"(w388) -> ()
        }
        frame #2 {
          # "LAB03"
          n227 = Concatenate Strings(w405, w396) -> (w406:string)
          n228 = String To Path(string=w406) -> (path=w404:path)
          n229 = Open/Create/Replace File(file path (use dialog)=w404, operation (0:open)=4) -> (refnum out=w403:refnum<file>, error out=w402:errorcluster)  [unwired: 4 in, 1 out]
          n230 = local read "LAB03 (CAL)"() -> (w397:T2)
          n231 = Write to Binary File(file (use dialog)=w403, data=w397, error in=w402) -> (refnum out=w401:refnum<file>, error out=w400:errorcluster)  [unwired: 3 in, 1 out]
          n232 = Close File(refnum=w401, error in=w400) -> (error out=w399:errorcluster)  [unwired: 1 out]
          n233 = local write "file error out"(w399) -> ()
        }
        frame #3 {
          # "LAB04"
          n234 = Concatenate Strings(w416, w407) -> (w417:string)
          n235 = String To Path(string=w417) -> (path=w415:path)
          n236 = Open/Create/Replace File(file path (use dialog)=w415, operation (0:open)=4) -> (refnum out=w414:refnum<file>, error out=w413:errorcluster)  [unwired: 4 in, 1 out]
          n237 = local read "LAB04 (CAL)"() -> (w408:T2)
          n238 = Write to Binary File(file (use dialog)=w414, data=w408, error in=w413) -> (refnum out=w412:refnum<file>, error out=w411:errorcluster)  [unwired: 3 in, 1 out]
          n239 = Close File(refnum=w412, error in=w411) -> (error out=w410:errorcluster)  [unwired: 1 out]
          n240 = local write "file error out"(w410) -> ()
        }
        frame #4 {
          # "LAB05"
          n241 = Concatenate Strings(w427, w418) -> (w428:string)
          n242 = String To Path(string=w428) -> (path=w426:path)
          n243 = Open/Create/Replace File(file path (use dialog)=w426, operation (0:open)=4) -> (refnum out=w425:refnum<file>, error out=w424:errorcluster)  [unwired: 4 in, 1 out]
          n244 = local read "LAB05 (CAL)"() -> (w419:T2)
          n245 = Write to Binary File(file (use dialog)=w425, data=w419, error in=w424) -> (refnum out=w423:refnum<file>, error out=w422:errorcluster)  [unwired: 3 in, 1 out]
          n246 = Close File(refnum=w423, error in=w422) -> (error out=w421:errorcluster)  [unwired: 1 out]
          n247 = local write "file error out"(w421) -> ()
        }
        frame #5 {
          # "TEMP REF"
          n248 = Concatenate Strings(w438, "T-REF-cal.bin") -> (w439:string)
          n249 = String To Path(string=w439) -> (path=w437:path)
          n250 = Open/Create/Replace File(file path (use dialog)=w437, operation (0:open)=4) -> (refnum out=w436:refnum<file>, error out=w435:errorcluster)  [unwired: 4 in, 1 out]
          n251 = local read "TEMP REF cal"() -> (w430:dbl)
          n252 = Write to Binary File(file (use dialog)=w436, data=w430, error in=w435) -> (refnum out=w434:refnum<file>, error out=w433:errorcluster)  [unwired: 3 in, 1 out]
          n253 = Close File(refnum=w434, error in=w433) -> (error out=w432:errorcluster)  [unwired: 1 out]
          n254 = local write "file error out"(w432) -> ()
        }
      }
    }
  }
